vi "Debug.vi"(8 "error in (no error)":errorcluster, 10 "Log Text":string, 11 "Logger in":refnum<class "Logger.lvclass">) -> (0 "error out":errorcluster, 3 "Logger out":refnum<class "Logger.lvclass">)   [LabVIEW 2020, in "LV Log.lvlib"]
uses:
  LV Log.lvlib
  Logger/Logger.lvclass
panel:
  out "Log Output":string
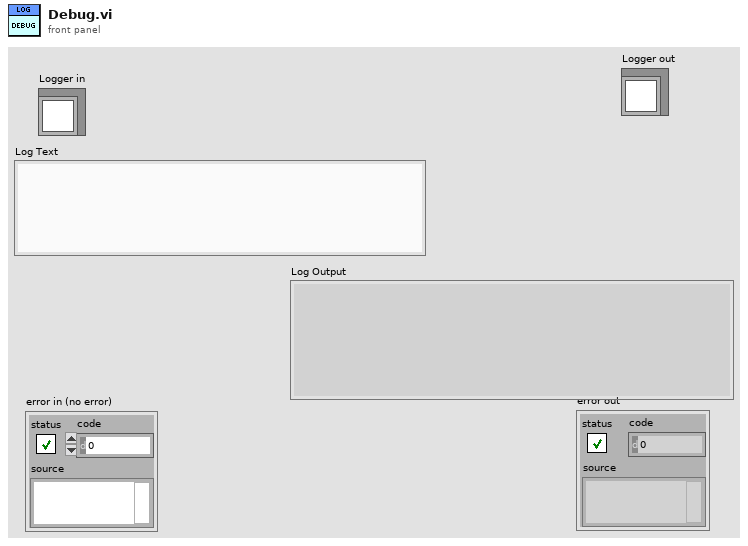
[diagram p1: front panel]
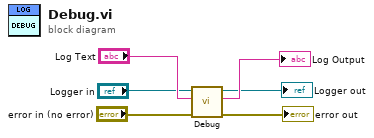
[diagram p0: block diagram]
diagram:
  n1 = call "Debug.vi"("error in (no error)"="error in (no error)", "Log Text"="Log Text", "Logger in"="Logger in") -> ("error out"=→"error out":errorcluster, "Log Output"=→"Log Output":string, "Logger out"=→"Logger out":refnum<class "Logger.lvclass">)  [unwired: 6 in]
